vi "PSDEV_Device Read Config.vi"(8 "error in":errorcluster caption="错误输入（无错误）") -> (0 "error out":errorcluster caption="错误输出", 2 "Succeed?":bool, 3 "Card":T1={"Module Type"="", "Module Name"="", "ModuSN"="", "ModuIP"="", "Used?"=FALSE, "Connected"=FALSE, "Timing*"={"Sample Rate"=1000.0}, "Channels"=[]})   [LabVIEW 2016]
uses:
  DAQ-Config/Controls/PSCHN_Channel Para.ctl
  DAQ-Config/Controls/PSCHN_Card Para.ctl
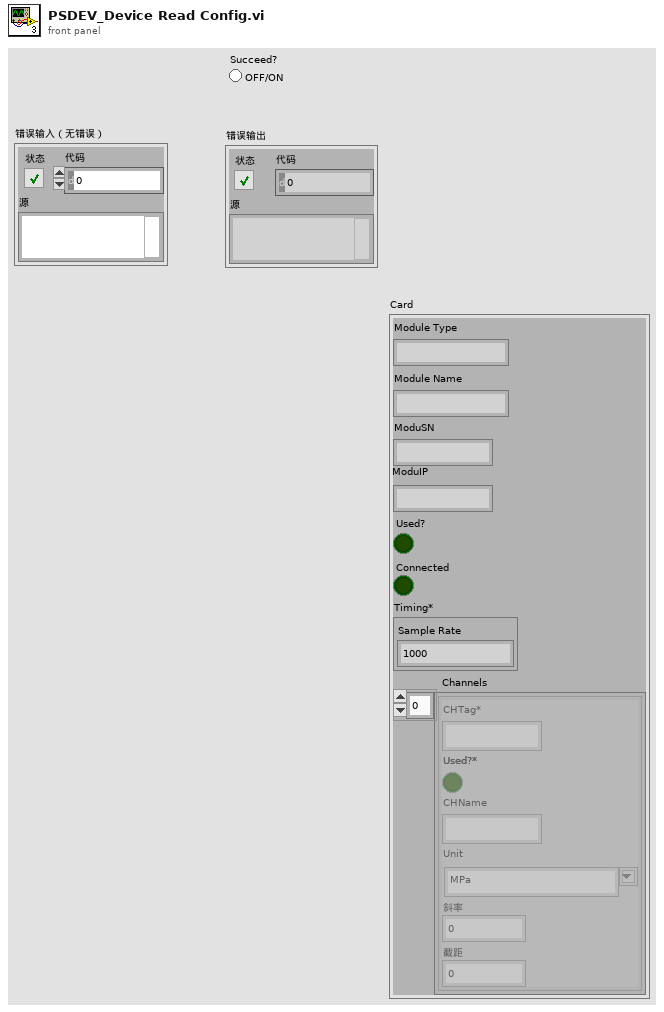
[diagram p1: front panel]
types:
  T1 = typedef "PSCHN_Card Para.ctl" = cluster{"Module Type":string, "Module Name":string, "ModuSN":string, "ModuIP":string, "Used?":bool, "Connected":bool, "Timing*":cluster{"Sample Rate":dbl}, "Channels":T2[]}
  T2 = typedef "PSCHN_Channel Para.ctl" = cluster{"CHTag*":string, "Used?*":bool, "CHName":string, "Unit":string, "斜率":dbl, "截距":dbl}
  T3 = cluster{"TREE PNG":path, "User Guide":path, "DefaultSave":path, "BuildPath":path, "Image":path, "Modules":path, "Configuration":path, "License":path, "SplitFiles":path, "System.ini":path}
  T4 = typedef "PSCHN_Card Para.ctl" = cluster{"Module Type":string, "Module Name":string, "Timing*":cluster{"Sample Rate":dbl, "Sample Mode*":i32, "Sample Time*":dbl, "Sample Speed*":u16}, "Used?":bool, "Channels":T5[], "Device":T8}
  T5 = typedef "PSCHN_Channel Para.ctl" = cluster{"Channel Name*":string, "Used?*":bool, "Assign Name":string, "Save?*":bool, "Range":dbl, "Unit*":string, "Scale Para*":T6, "Scale Result":string, "Channel Data*":variant, "Measurement Type*":T7, "斜率*":dbl, "截距*":dbl, "Electrical Zero":dbl, "Electrical Sensitivity":dbl, "Physical Zero*":dbl, "Physical Nominal":dbl, "Output rate*":dbl, "User Signal ID*":i32, "UUID*":string, "Connector number*":i32}
  T6 = typedef "Scale DS.ctl" = cluster{"Scale Name*":string, "ScaleType*":i32, "Pre-Units*":i32, "Scaled Units":string, "Value*":variant}
  T7 = typedef "PSDAN_Measurement Type.ctl" = u16
  T8 = typedef "QX_DeviceType.ctl" = cluster{"UUID":string, "Port":i32, "IP":string, "No Of Chans":i32, "Name":string}
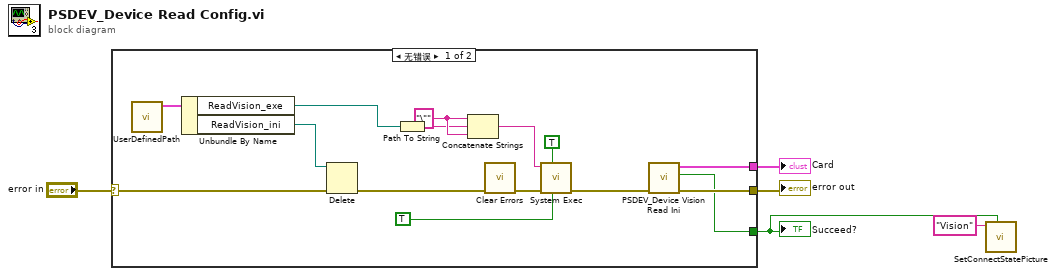
[diagram p0: block diagram]
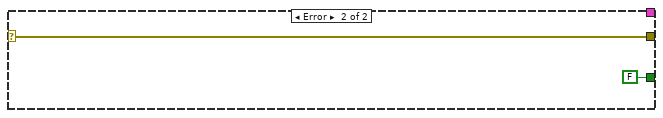
[diagram p2: hidden frame]
diagram:
  n1 = case shown="无错误" "error in" {
    selector: "error in" -> [w10 w22]
    tunnel: [w8 w22] -> w5
    tunnel: [w7 _] -> w3
    tunnel: [w6 FALSE ("Succeed?")] -> w2
    frame No Error {
      w17 = "\"" ("String")
      n2 = call "UserDefinedPath.vi"() -> ("UserDefinedPath"=w14:T3)  [unwired: 11 in]
      n3 = Unbundle By Name(w14) -> ("ReadVision_exe"=w13:path, "ReadVision_ini"=w12:path)
      n4 = Delete(path (use dialog)=w12, error in=w10) -> (error out=w11:errorcluster)  [unwired: 3 in, 2 out]
      n5 = Path To String(path=w13) -> (string=w16:string)
      n6 = Concatenate Strings(w17, w16, w17) -> (w18:string)
      n7 = call <vilib>:"Clear Errors.vi"("error in (no error)"=w11) -> ("error out"=w19:errorcluster)  [unwired: 5 in, 1 out]
      n8 = call <vilib>:"System Exec.vi"("run minimized? (F)"=TRUE, "wait until completion? (T)"=TRUE, "error in (no error)"=w19, "command line"=w18) -> ("error out"=w9:errorcluster)  [unwired: 4 in, 3 out]
      n9 = call "PSDEV_Device Vision Read Ini.vi"("error in"=w9) -> ("error out"=w8:errorcluster, "Succeed?"=w6:bool, "Card"=w7:T4)  [unwired: 8 in]
    }
    frame Error {
    }
  }
  "error out" <- w5
  "Card" <- w3
  "Succeed?" <- w2
  n10 = call "SetConnectStatePicture.vi"("connected?"=w2, "活动项:标识符"="Vision") -> ()  [unwired: 10 in]
